vi "Read Config File.vi"(0 "Config File Ref Num":T2, 1 "VI reference (current VI)":refnum<vi>, 5 "Standalone":bool=TRUE, 9 "file path (use dialog)":path, 11 "error in":errorcluster, 12 "All or partial":T1(ring)=enum."Read Single Section", 13 "Keys to Create/Update":cluster{"Key Name":string, "Key Data":string}[](array[cluster]), 14 "section (read or create/update)":string) -> (4 "INI Data Out":T3(array[cluster]), 6 "section names":string[](array[string]), 8 "found?":bool, 10 "key names":string[](array[string]), 15 "error out":errorcluster)   [LabVIEW 2017]
uses:
  <vilib>/Utility/config.llb/Config Data RefNum.ctl
  <vilib>/Utility/config.llb/Read Key (String).vi
  <vilib>/Utility/config.llb/NI_LVConfig.lvlib
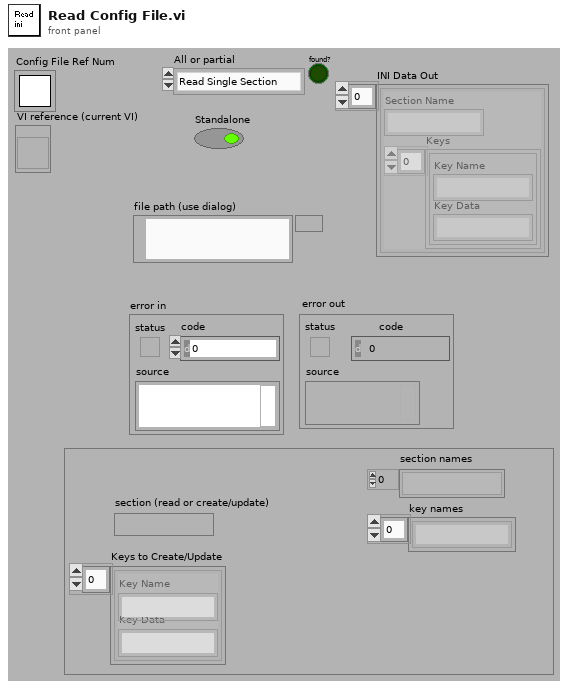
[diagram p1: front panel]
types:
  T1 = enum32{"Read All Sections", "Read Single Section", "Update All Sections", "Create/Update Section"}
  T2 = typedef "NI_LVConfig.lvlib/Config Data RefNum.ctl" = refnum<k1>
  T3 = cluster{"Section Name":string, "Keys":cluster{"Key Name":string, "Key Data":string}[]}[]
  T4 = cluster{"Section Name":string, "Keys":cluster{"Key Name":string, "Key Data":string}[]}
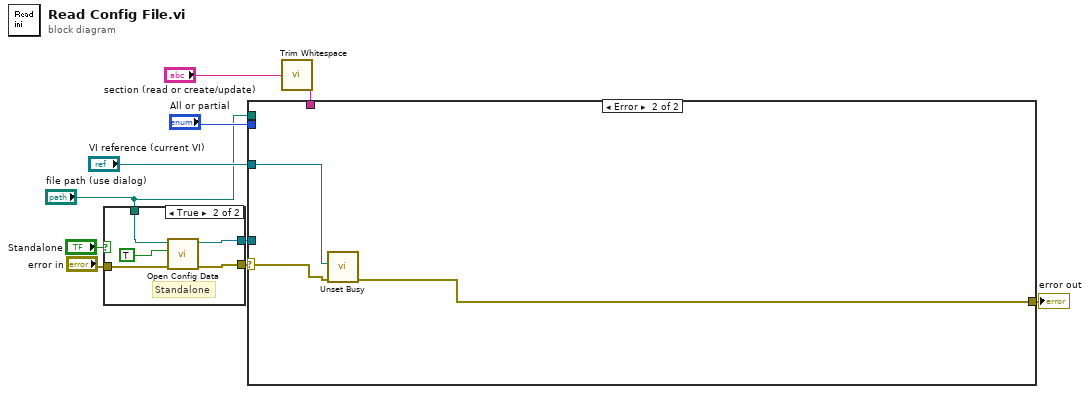
[diagram p0: block diagram]
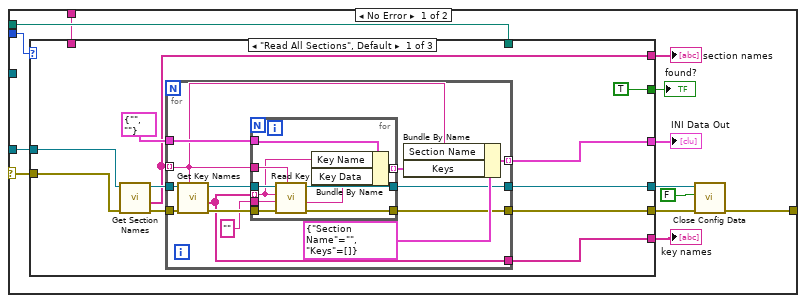
[diagram p2: hidden frame]
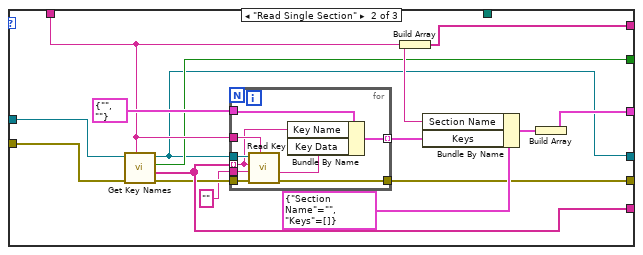
[diagram p3: hidden frame]
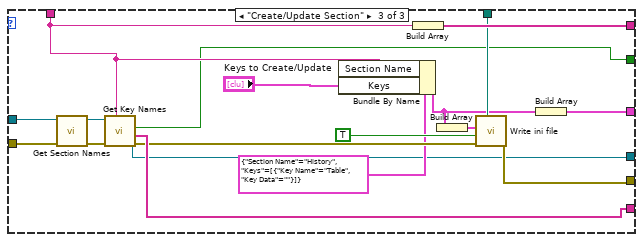
[diagram p4: hidden frame]
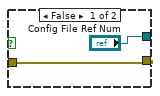
[diagram p5: hidden frame]
diagram:
  n1 = case shown="True" "Standalone" {
    tunnel: [w11 w17] -> w7
    tunnel: ["Config File Ref Num" w16] -> w8
    tunnel: "error in" -> [w11 w15]
    tunnel: "file path (use dialog)" -> [_ w13]
    frame False {
    }
    frame True {
      # "Standalone"
      n2 = call <vilib>:"Open Config Data.vi"("error in (no error)"=w15, "create file if necessary (T)"=TRUE ("create file if necessary? (T)"), "configuration file path"=w13) -> ("error out"=w17:errorcluster, "refnum"=w16:T2)  [unwired: 6 in, 1 out]
    }
  }
  n3 = call <vilib>:"Trim Whitespace.vi"("string"="section (read or create/update)") -> ("trimmed string"=w1:string)  [unwired: 1 in]
  n4 = case shown="Error" w7 {
    selector: w7 -> [w29 w109]
    tunnel: w8 -> [w30 _]
    tunnel: [w21 w108] -> w6
    tunnel: "VI reference (current VI)" -> [_ w107]
    tunnel: "All or partial" -> [w28 _]
    tunnel: "file path (use dialog)" -> [w24 _]
    tunnel: w1 -> [w23 _]
    frame No Error {
      n5 = case shown="\"Read All Sections\", Default" w28 {
        tunnel: w30 -> [w41 w72 w106]
        tunnel: w29 -> [w40 w71 w105]
        tunnel: [w33 w67 w92] -> w20
        tunnel: [w36 w70 w102] -> w27
        tunnel: [w35 w77 w101] -> w26
        tunnel: [w34 w68 w100] -> w25
        tunnel: w24 -> [_ _ w99]
        tunnel: w23 -> [_ w69 w98]
        tunnel: [w32 w65 w91] -> w19
        tunnel: [TRUE ("found?") w66 w89] -> w18
        frame "Read All Sections", Default {
          n6 = call <vilib>:"Get Section Names.vi"("error in (no error)"=w40, "refnum"=w41) -> ("error out"=w38:errorcluster, "section names"=w34:string[], "refnum out"=w39:T2)  [unwired: 7 in]
          n7 = for {
            tunnel: w34 -> [w46] mode=indexing
            tunnel: w39 -> [w54]
            tunnel: w38 -> [w53]
            tunnel: cluster{"Key Name":string, "Key Data":string} {"Key Name"="", "Key Data"=""} ("Keys") -> [w49]
            tunnel: [w45] -> w36 mode=indexing
            tunnel: [w44] -> w32
            tunnel: [w43] -> w33
            tunnel: [w42] -> w35
            n8 = call <vilib>:"Get Key Names.vi"("section"=w46, "error in (no error)"=w53, "refnum"=w54) -> ("error out"=w51:errorcluster, "key names"=w42:string[], "refnum out"=w52:T2)  [unwired: 6 out]
            n9 = for {
              tunnel: w52 -> [w64]
              tunnel: w46 -> [w63]
              tunnel: w42 -> [w57] mode=indexing
              tunnel: w51 -> [w62]
              tunnel: "" -> [w61]
              tunnel: [w60] -> w44
              tunnel: [w59] -> w43
              tunnel: w49 -> [w56]
              tunnel: [w55] -> w47 mode=indexing
              n10 = call-poly <vilib>:"Read Key.vi"("section"=w63, "error in (no error)"=w62, "default value"=w61, "key"=w57, "refnum"=w64) -> ("error out"=w59:errorcluster, "value"=w58:string, "refnum out"=w60:T2)  [unwired: 1 in, 3 out]
              n11 = Bundle By Name(cluster=w56, "Key Name"=w57, "Key Data"=w58) -> (w55:cluster{"Key Name":string, "Key Data":string})
            }
            n12 = Bundle By Name(cluster=T4 {"Section Name"="", "Keys"=[]} ("Key Data"), "Section Name"=w46, "Keys"=w47) -> (w45:T4)
          }
        }
        frame "Read Single Section" {
          n13 = call <vilib>:"Get Key Names.vi"("section"=w69, "error in (no error)"=w71, "refnum"=w72) -> ("error out"=w76:errorcluster, "key names"=w77:string[], "section exists?"=w66:bool, "refnum out"=w65:T2)  [unwired: 5 out]
          n14 = for {
            tunnel: w65 -> [w88]
            tunnel: w69 -> [w87]
            tunnel: w77 -> [w82] mode=indexing
            tunnel: w76 -> [w86]
            tunnel: "" -> [w85]
            tunnel: [w84] -> w67
            tunnel: cluster{"Key Name":string, "Key Data":string} {"Key Name"="", "Key Data"=""} ("Keys") -> [w81]
            tunnel: [w80] -> w73 mode=indexing
            n15 = call-poly <vilib>:"Read Key.vi"("section"=w87, "error in (no error)"=w86, "default value"=w85, "key"=w82, "refnum"=w88) -> ("error out"=w84:errorcluster, "value"=w83:string)  [unwired: 1 in, 4 out]
            n16 = Bundle By Name(cluster=w81, "Key Name"=w82, "Key Data"=w83) -> (w80:cluster{"Key Name":string, "Key Data":string})
          }
          n17 = Build Array(w69) -> (w68:string[])
          n18 = Bundle By Name(cluster=T4 {"Section Name"="", "Keys"=[]} ("Key Data"), "Section Name"=w69, "Keys"=w73) -> (w78:T4)
          n19 = Build Array(w78) -> (w70:T3)
        }
        frame "Create/Update Section" {
          n20 = call <vilib>:"Get Section Names.vi"("error in (no error)"=w105, "refnum"=w106) -> ("error out"=w103:errorcluster, "refnum out"=w104:T2)  [unwired: 7 in, 1 out]
          n21 = call <vilib>:"Get Key Names.vi"("section"=w98, "error in (no error)"=w103, "refnum"=w104) -> ("error out"=w97:errorcluster, "key names"=w101:string[], "section exists?"=w89:bool, "refnum out"=w91:T2)  [unwired: 5 out]
          n22 = Bundle By Name(cluster=T4 {"Section Name"="History", "Keys"=[{"Key Name"="Table", "Key Data"=""}]} ("Key Data"), "Section Name"=w98, "Keys"="Keys to Create/Update") -> (w96:T4)
          n23 = Build Array(w98) -> (w100:string[])
          n24 = Build Array(w96) -> (w93:T3)
          n25 = call "Write ini file.vi"("file path (use dialog)"=w99, "error in"=w97, "Standalone?"=TRUE, "INI Data"=w93) -> ("error out"=w92:errorcluster)  [unwired: 3 in, 4 out]
          n26 = Build Array(w96) -> (w102:T3)
        }
      }
      "found?" <- w18
      "INI Data Out" <- w27
      "key names" <- w26
      "section names" <- w25
      n27 = call <vilib>:"Close Config Data.vi"("error in (no error)"=w20, "write file if changed (T)"=FALSE ("write configuration file? (T)"), "refnum"=w19) -> ("error out"=w21:errorcluster)  [unwired: 8 out]
    }
    frame Error {
      n28 = call <vilib>:"Unset Busy.vi"("error in (no error)"=w109, "VI reference (current VI)"=w107) -> ("error out"=w108:errorcluster)  [unwired: 9 out]
    }
  }
  "error out" <- w6
